vi "Create File for Gear SS.vi"() -> (2 "File Reference Out":refnum<file>)   [LabVIEW 2016]
uses:
  Global Variables/Folder Names.vi
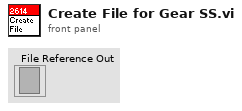
[diagram p1: front panel]
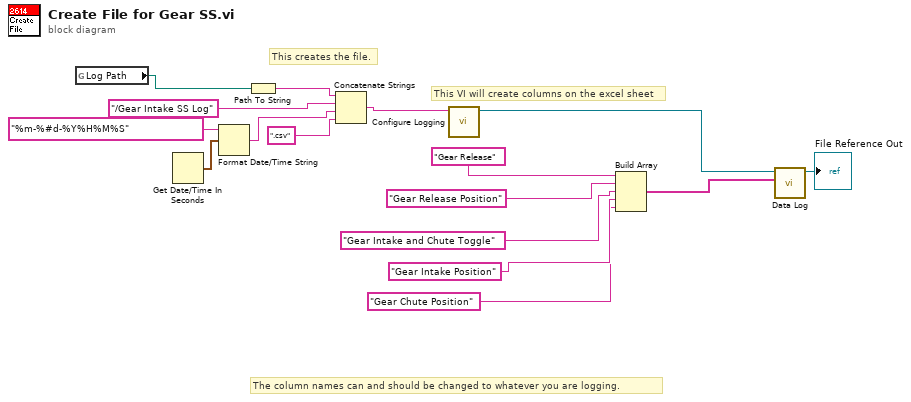
[diagram p0: block diagram]
diagram:
  # "The column names can and should be changed to whatever you are logging."
  # "This VI will create columns on the excel sheet"
  # "This creates the file."
  n1 = global read "Folder Names.vi" "Log Path"() -> (w14:path)
  n2 = Get Date/Time In Seconds() -> (seconds since 1Jan1904=w8:timestamp)
  n3 = Format Date/Time String(time format string (%c)="%m-%#d-%Y%H%M%S", seconds (now)=w8) -> (date/time string=w6:string)  [unwired: 1 in]
  n4 = Path To String(path=w14) -> (string=w13:string)
  n5 = Concatenate Strings(w13, "/Gear Intake SS Log" ("string"), w6, ".csv" ("string")) -> (w15:string)
  n6 = call "Configure Logging.vi"("File Path/File Name"=w15) -> ("refnum out"=w10:refnum<file>)  [unwired: 10 in]
  n7 = Build Array("Gear Release" ("File Path/File Name"), "Gear Release Position" ("File Path/File Name"), "Gear Intake and Chute Toggle" ("File Path/File Name"), "Gear Intake Position" ("File Path/File Name"), "Gear Chute Position" ("element")) -> (w12:string[])
  n8 = call "Data Log.vi"("Data In"=w12, "File Reference In"=w10) -> ("File Reference Out"=→"File Reference Out":refnum<file>)  [unwired: 9 in]
